vi "version nos.vi"() -> ()   [LabVIEW 2018, in "LV-0mq-Julia_roundtrip-lib.lvlib"]
uses:
  LV-0mq-Julia_roundtrip-lib.lvlib
  VersionNumber.ctl
panel:
  in  "Pkg version":T1={"major"=0, "minor"=1, "patch"=1}
  out "PROTOC_V":u8=1
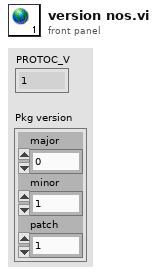
[diagram p1: front panel]
types:
  T1 = typedef "LV-0mq-Julia_roundtrip-lib.lvlib/VersionNumber.ctl" = cluster{"major":u16, "minor":u16, "patch":u16}
diagram:
